vi "Request TimerUserEvent.vi"(8 "error in (no error)":errorcluster, 10 "TimePeroid(ms)":i64, 11 "TimerEngine in":refnum<class "TimerEngine.lvclass">) -> (0 "error out":errorcluster, 1 "TimerUserEvent":T1, 2 "TimePeroid(ms) OUT":i64, 3 "TimerEngine out":refnum<class "TimerEngine.lvclass">)   [LabVIEW 2017, in "TimerEngine.lvlib" / "TimerEngine.lvclass"]
uses:
  TimerEngine.lvclass
  _Typedef/Timer-UserEvent.ctl
  TimerEngine.lvclass/TimerEngine.ctl
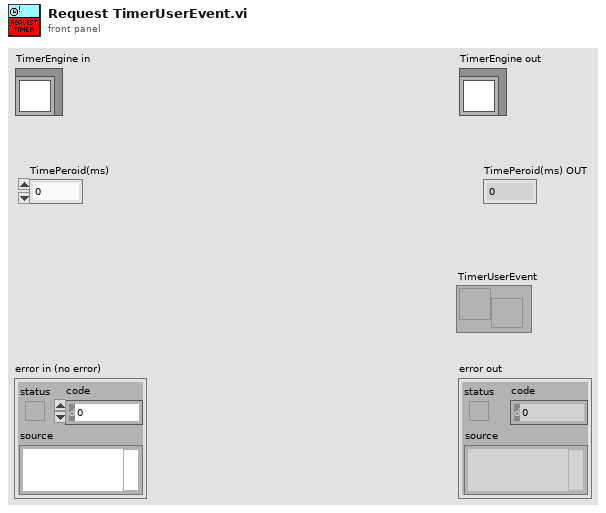
[diagram p1: front panel]
types:
  T1 = typedef "TimerEngine.lvlib/TimerEngine.lvclass/Timer-UserEvent.ctl" = refnum<user-event>
  T2 = typedef "TimerEngine.lvlib/TimerEngine.lvclass/WatchDog--QueueRef.ctl" = refnum<queue>
  T3 = cluster{"TimePeroid(ms)":i64, "queue out":refnum<queue>, "TimerEngine in":refnum<class "TimerEngine.lvclass">}
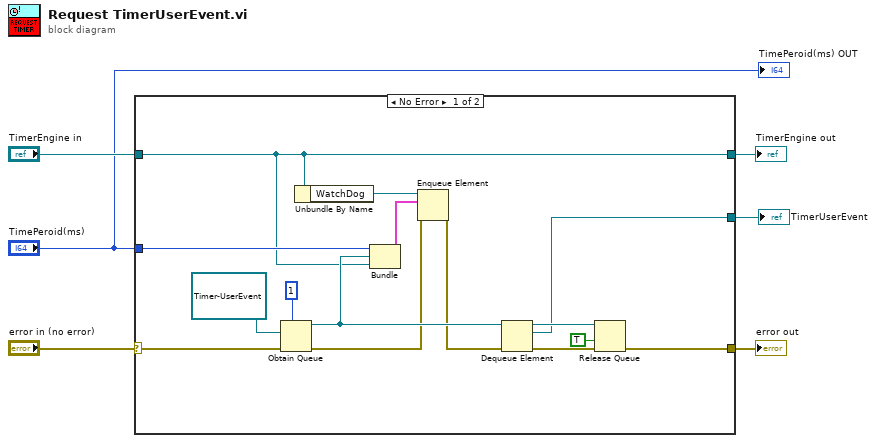
[diagram p0: block diagram]
diagram:
  n1 = case shown="No Error" "error in (no error)" {
    selector: "error in (no error)" -> [w14 w23]
    tunnel: [w12 w23] -> w5
    tunnel: [w7 w22] -> w3
    tunnel: "TimerEngine in" -> [w7 w22]
    tunnel: "TimePeroid(ms)" -> [w20 _]
    tunnel: [w8 _] -> w2
    frame No Error {
      n2 = Obtain Queue(max queue size (-1, unlimited)=1, element data type=T1 refnum ("UserEvent"), error in (no error)=w14) -> (queue out=w16:refnum<queue>, error out=w10:errorcluster)  [unwired: 2 in, 1 out]
      n3 = Unbundle By Name(w7) -> ("WatchDog"=w21:T2)
      n4 = Bundle("TimePeroid(ms)"=w20, "queue out"=w16, "TimerEngine in"=w7) -> (w17:T3)  [unwired: 1 in]
      n5 = Enqueue Element(queue=w21, element=w17, error in (no error)=w10) -> (error out=w9:errorcluster)  [unwired: 1 in, 2 out]
      n6 = Dequeue Element(queue=w16, error in (no error)=w9) -> (queue out=w15:refnum<queue>, element=w8:T1, error out=w13:errorcluster)  [unwired: 1 in, 1 out]
      n7 = Release Queue(queue=w15, force destroy? (F)=TRUE, error in (no error)=w13) -> (error out=w12:errorcluster)  [unwired: 2 out]
    }
    frame Error {
    }
  }
  "error out" <- w5
  "TimerEngine out" <- w3
  "TimerUserEvent" <- w2
  "TimePeroid(ms) OUT" <- "TimePeroid(ms)"
